vi "Light321.vi"(3 "error in (no error)":errorcluster, 5 "VISA resource name":refnum<visa-resource-name>) -> (0 "error out":errorcluster, 2 "VISA resource name out":refnum<visa-resource-name>)   [LabVIEW 2009]
doc: "Flashes the light on a cyberglove in a 3...2...1 (flashes) pattern. Can be used as a countdown of sorts."
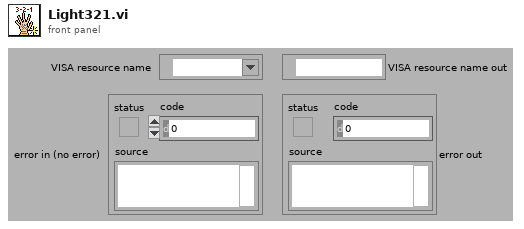
[diagram p1: front panel]
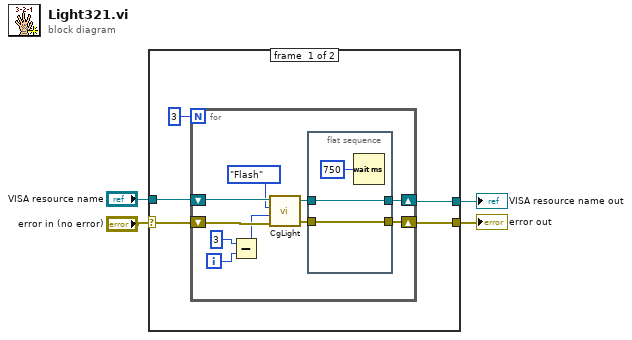
[diagram p0: block diagram]
diagram:
  n1 = case shown="No Error" "error in (no error)" {
    selector: "error in (no error)" -> [w7 w24]
    tunnel: [w8 w24] -> w3
    tunnel: "VISA resource name" -> [w6 w23]
    tunnel: [w5 w23] -> w1
    frame #0 {
      n2 = for {
        N: 3 -> [_]
        shift-right: [w10] -> w5
        shift-left: w6 -> [w19]
        shift-right: [w11] -> w8
        shift-left: w7 -> [w18]
        i -> [w16]
        n3 = Subtract(x=3, y=w16) -> (x-y=w14:i32)
        n4 = call "CgLight.vi"("error in (no error)"=w18, "Flashes"=w14, "Mode"=enum16{"Off", "On", "Flash"}."Flash", "VISA resource name"=w19) -> ("error out"=w12:errorcluster, "VISA resource name out"=w13:refnum<visa-resource-name>)  [unwired: 1 in]
        n5 = flat-sequence {
          tunnel: w13 -> [w20]
          tunnel: w12 -> [w21]
          tunnel: [w21] -> w11
          tunnel: [w20] -> w10
          frame #0 {
            n6 = Wait (ms)(milliseconds to wait=u32 750) -> ()  [unwired: 1 out]
          }
        }
      }
    }
    frame #1 {
    }
  }
  "error out" <- w3
  "VISA resource name out" <- w1
